vi "Uim ACK wrapper.vi"(8 "error in (no error)":errorcluster caption="错误输入（无错误）", 10 "dwCanNodeId":u32, 11 "dwDevIndex":u32) -> (0 "error out":errorcluster caption="错误输出", 1 "BASIC_ACK_OBJ":T1, 3 "function return":u32)   [LabVIEW 2016, in "UISimCanFunc_wrapper.lvlib"]
doc: "_declspec (dllexport) DWORD UimACK_wrapper(DWORD dwDevIndex, DWORD dwCanNodeId, P_BASIC_ACK_OBJ pACKInfo);"
uses:
  <userlib>/UISimCanFunc_wrapper/UISimCanFunc_wrapper.lvlib
  <userlib>/UISimCanFunc_wrapper/ctl/BASIC_ACK_OBJ.ctl
  <userlib>/UISimCanFunc_wrapper/UISimCanFunc_wrapper.dll
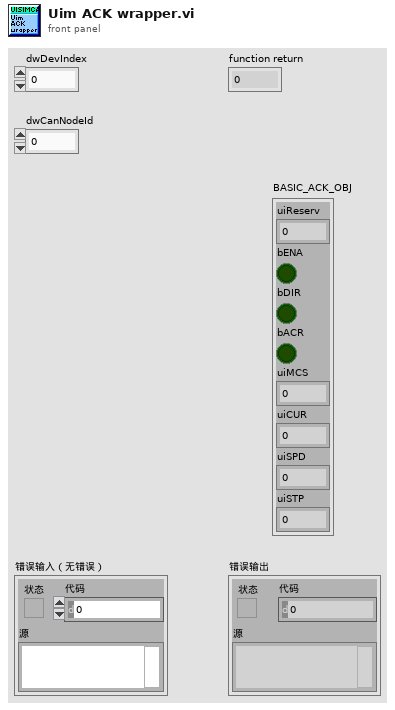
[diagram p1: front panel]
types:
  T1 = typedef "UISimCanFunc_wrapper.lvlib/BASIC_ACK_OBJ.ctl" = cluster{"uiReserv":u32, "bENA":bool, "bDIR":bool, "bACR":bool, "uiMCS":u32, "uiCUR":u32, "uiSPD":u32, "uiSTP":u32}
  T2 = cluster{"uiReserv":u32, "bENA":i32, "bDIR":i32, "bACR":i32, "uiMCS":u32, "uiCUR":u32, "uiSPD":u32, "uiSTP":u32}
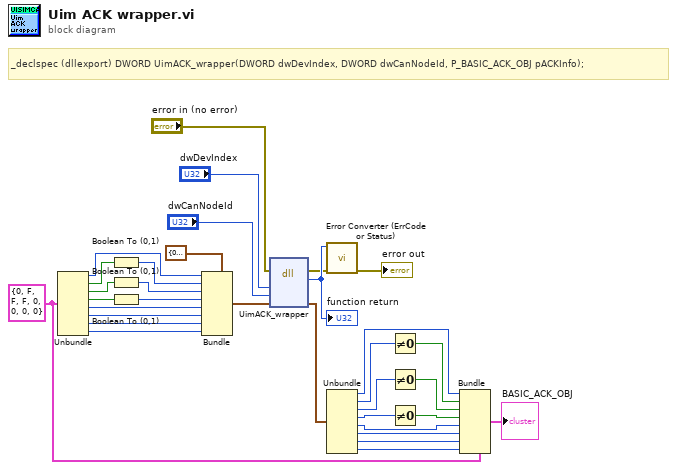
[diagram p0: block diagram]
diagram:
  w13 = T1 {"uiReserv"=0, "bENA"=FALSE, "bDIR"=FALSE, "bACR"=FALSE, "uiMCS"=0, "uiCUR"=0, "uiSPD"=0, "uiSTP"=0} ("BASIC_ACK_OBJ")
  # "_declspec (dllexport) DWORD UimACK_wrapper(DWORD dwDevIndex, DWORD dwCanNodeId, P_BASIC_ACK_OBJ pACKInfo);"
  n1 = Unbundle(w13) -> ("uiReserv"=w25:u32, "bENA"=w24:bool, "bDIR"=w23:bool, "bACR"=w22:bool, "uiMCS"=w18:u32, "uiCUR"=w17:u32, "uiSPD"=w16:u32, "uiSTP"=w15:u32)
  n2 = Boolean To (0,1)(Boolean=w24) -> (0, 1=w21:i16)
  n3 = Boolean To (0,1)(Boolean=w23) -> (0, 1=w20:i16)
  n4 = Boolean To (0,1)(Boolean=w22) -> (0, 1=w19:i16)
  n5 = Bundle(cluster=T2 {"uiReserv"=0, "bENA"=0, "bDIR"=0, "bACR"=0, "uiMCS"=0, "uiCUR"=0, "uiSPD"=0, "uiSTP"=0} ("pACKInfo"), "uiReserv"=w25, "bENA"=w21, "bDIR"=w20, "bACR"=w19, "uiMCS"=w18, "uiCUR"=w17, "uiSPD"=w16, "uiSTP"=w15) -> (w26:T2)
  n6 = dll-call lib="C:/Program Files (x86)/National Instruments/LabVIEW 2016/user.lib/UISimCanFunc_wrapper/UISimCanFunc_wrapper.*" fn="UimACK_wrapper"(error in="error in (no error)", "dwDevIndex"="dwDevIndex", "dwCanNodeId"="dwCanNodeId", "pACKInfo"=w26) -> (error out=w29:errorcluster, w33:u32, "pACKInfo"=w14:T2)  [unwired: 4 in, 1 out]
  "function return" <- w33
  n7 = call <userlib>:"Error Converter (ErrCode or Status).vi"("error in (no error)"=w29, "error code"=w33) -> ("error out"=→"error out":errorcluster)  [unwired: 9 in]
  n8 = Unbundle(w14) -> ("uiReserv"=w12:u32, "bENA"=w11:i32, "bDIR"=w10:i32, "bACR"=w9:i32, "uiMCS"=w5:u32, "uiCUR"=w4:u32, "uiSPD"=w3:u32, "uiSTP"=w2:u32)
  n9 = Not Equal To 0?(x=w11) -> (x != 0?=w8:bool)
  n10 = Not Equal To 0?(x=w10) -> (x != 0?=w7:bool)
  n11 = Not Equal To 0?(x=w9) -> (x != 0?=w6:bool)
  n12 = Bundle(cluster=w13, "uiReserv"=w12, "bENA"=w8, "bDIR"=w7, "bACR"=w6, "uiMCS"=w5, "uiCUR"=w4, "uiSPD"=w3, "uiSTP"=w2) -> (→"BASIC_ACK_OBJ":T1)
